vi "Write Path.vi"(8 "error in (no error)":errorcluster, 10 "Path":path, 11 "Text Actor in":refnum<class "Text Actor.lvclass">) -> (0 "error out":errorcluster, 3 "Text Actor out":refnum<class "Text Actor.lvclass">)   [LabVIEW 2020, in "Text Actor.lvlib" / "Text Actor.lvclass"]
uses:
  Text Actor.lvclass
  Text Actor.lvclass/Text Actor.ctl
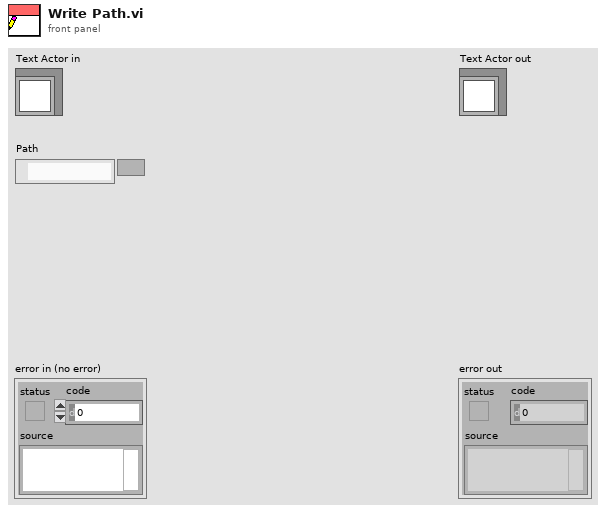
[diagram p1: front panel]
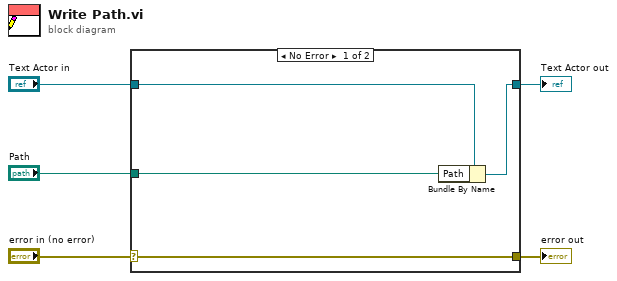
[diagram p0: block diagram]
diagram:
  n1 = case shown="No Error" "error in (no error)" {
    selector: "error in (no error)" -> [w9 w10]
    tunnel: [w9 w10] -> w4
    tunnel: [w7 w11] -> w2
    tunnel: "Text Actor in" -> [w8 w11]
    tunnel: "Path" -> [w6 _]
    frame No Error {
      n2 = Bundle By Name(cluster=w8, "Path"=w6) -> (w7:refnum<class "Text Actor.lvclass">)
    }
    frame Error {
    }
  }
  "error out" <- w4
  "Text Actor out" <- w2
